vi "VL53L0X_SetLimitCheckEnableSigmaFinalRange.vi"(6 "enable (T)":bool=TRUE, 9 "addr":i32, 10 "?":T1, 11 "error in (no error)":errorcluster) -> (2 "Status":bool, 3 "error out":errorcluster)   [LabVIEW 2019, in "DistanceSensorDriver.lvlib"]
uses:
  DistanceSensorDriver.lvlib
  Typedef/Ports.ctl
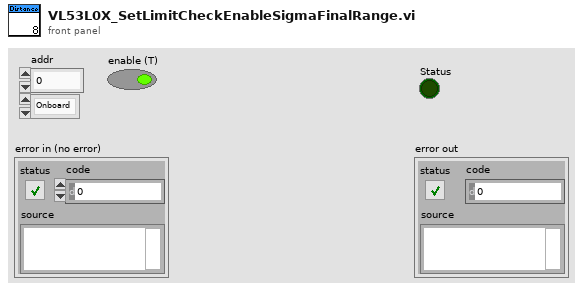
[diagram p1: front panel]
types:
  T1 = typedef "DistanceSensorDriver.lvlib/Ports.ctl" = enum32{"Onboard", "MXP"}
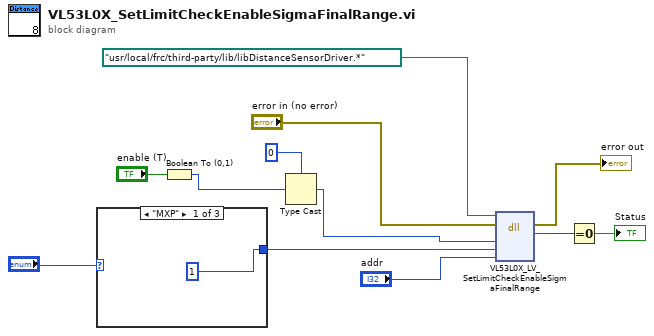
[diagram p0: block diagram]
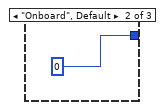
[diagram p2: hidden frame]
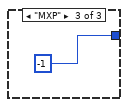
[diagram p3: hidden frame]
diagram:
  n1 = case shown="\"MXP\"" "?" {
    tunnel: [1 ("port") 0 ("port") -1 ("port")] -> w9
    frame "MXP" {
    }
    frame "Onboard", Default {
    }
    frame "MXP" {
    }
  }
  n2 = Boolean To (0,1)(Boolean="enable (T)") -> (0, 1=w3:i16)
  n3 = Type Cast(type=0, x=w3) -> (*(type *) &x=w1:i32)
  n4 = dll-call lib="?" fn="VL53L0X_LV_SetLimitCheckEnableSigmaFinalRange"(path in=path "/usr/local/frc/third-party/lib/libDistanceSensorDriver.*", error in="error in (no error)", "enable"=w1, "port"=w9, "addr"="addr") -> (error out=→"error out":errorcluster, "return type"=w8:i32)  [unwired: 4 in, 1 out]
  n5 = Equal To 0?(x=w8) -> (x = 0?=→"Status":bool)
